vi "Process.vi"(8 "error in":errorcluster, 11 "Instrument.Example":refnum<class "Instrument.OxfordVRM.lvclass">) -> (0 "error out":errorcluster, 3 "Instrument.Example out":refnum<class "Instrument.OxfordVRM.lvclass">)   [LabVIEW 2019, in "Instrument.OxfordVRM.lvclass"]
doc: "---------------------------------------------------------------\nJKI State Machine Objects™\nhttp://jki.net/state-machine-objects/\nCopyright (C) 2005-2015, JKI <info@jki.net>\nALL RIGHTS RESERVED"
uses:
  Instrument.OxfordVRM.lvclass
  C:/Program Files (x86)/National Instruments/LabVIEW 2019/vi.lib/JKI/JKI SMO/SMO/SMO.lvclass
  C:/Program Files (x86)/National Instruments/LabVIEW 2019/user.lib/LevyLab/Instrument Framework/Instrument/Instrument.lvclass
  Typedefs/VRM Magnet Axis--Enum.ctl
  Instrument.OxfordVRM.lvclass/Instrument.OxfordVRM.ctl
  <vilib>/JKI/JKI SMO/SMO/SMO.lvclass/SMO.ctl
  <vilib>/JKI/JKI SMO/SMO/Private/ReftoDVR--SMO.vi
  <userlib>/LevyLab/Instrument Framework/Instrument Types/Cryostat/Instrument.Cryostat.lvclass
  <vilib>/JKI/JKI SMO/SMO/SMO.lvclass
  <userlib>/LevyLab/Instrument Framework/Instrument/Instrument.lvclass
  <userlib>/LevyLab/Debug/Debug.lvlib
panel:
  out "State":string
  out "timer":u32
  # "For instructions on how to use the JKI State Machine Objects, examples and video tutorials, visit:\nhttp://jki.net/state-machine-objects/\n\nJKI State Machine Objects™\nhttp://jki.net/state-machine-objects/\nCopyright (C) 2005-2015, JKI <info@jki.net>\nALL RIGHTS RESERVED"
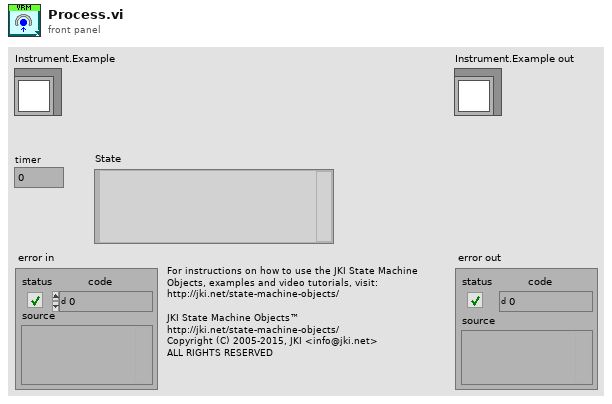
[diagram p1: front panel]
types:
  T1 = enum32{"invalid app kind", "Development System", "Run Time System", "Student Edition", "Embedded LabVIEW", "Evaluation", "Custom"}
  T2 = enum32{"Invalid", "Standard", "Closed", "Hidden", "Minimized", "Maximized"}
  T3 = typedef "Instrument.OxfordVRM.lvclass/VRM Magnet Axis--Enum.ctl" = enum16{"X", "Y", "Z", "ALL"}
  T4 = cluster{"Core":cluster{"Current VI Reference":refnum<vi>, "Close Panel on Exit?":bool, "Last Error":cluster{"error":errorcluster, "previous state":string, "remaining states":string}, "Shutdown?":bool}, "SelfRef":refnum<class "Instrument.OxfordVRM.lvclass">, "Field (T)":dbl[], "Field Rate (T/min)":dbl, "Axis":T3, "Running Step":i32, "sequence":string[]}
  T5 = cluster{"Current VI Reference":refnum<vi>, "Close Panel on Exit?":bool, "Last Error":cluster{"error":errorcluster, "previous state":string, "remaining states":string}, "Shutdown?":bool}
  T6 = typedef "Instrument.OxfordVRM.lvclass/getAll.ctl" = cluster{"Field":dbl[], "Target Field":dbl[], "Target Field Rate":dbl[], "PSU Current":dbl[], "PSU Voltage":dbl[], "Status":string[]}
  T7 = typedef "Debug.lvlib/Attribute.Debug.lvclass/DebugBehavior.ctl" = enum16{"Normal", "Debug"}
  T8 = typedef "SMO.lvclass/Protected Events.ctl" = cluster{"StopProcesses":refnum<user-event>, "AbortProcesses":refnum<user-event>, "Config Changed":refnum<user-event>, "Dependency":refnum<user-event>}
  T9 = typedef "Instrument.OxfordVRM.lvclass/PrivateEvents--Cluster.ctl" = cluster{"SequenceSetMagnetField":refnum<user-event>, "AbortSequence":refnum<user-event>}
  T10 = cluster{"Holding":bool, "Ramp to Setpoint":bool, "Ramp to Zero":bool, "Clamp":bool}
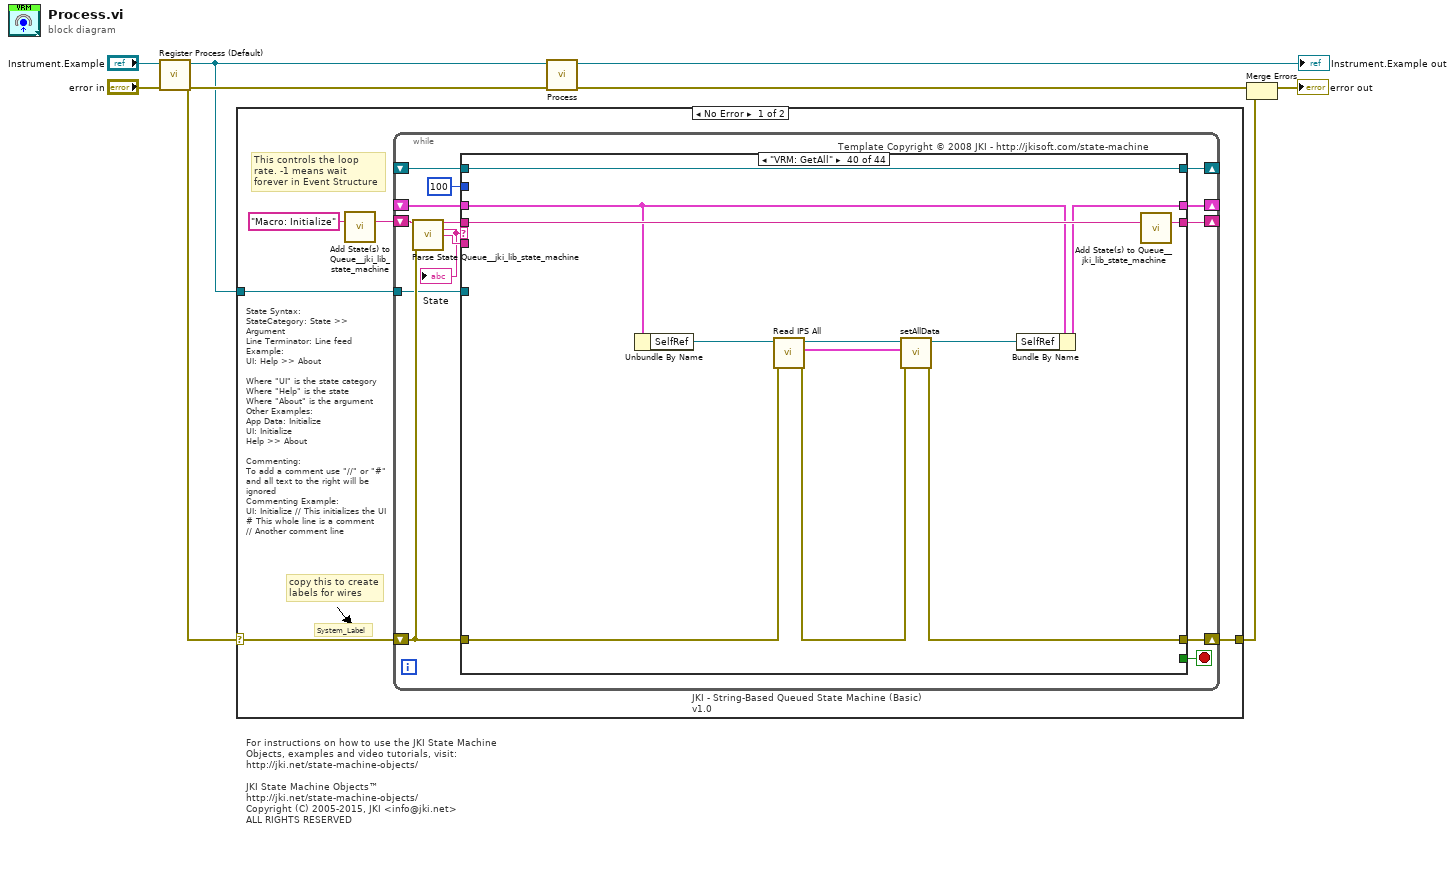
[diagram p0: block diagram]
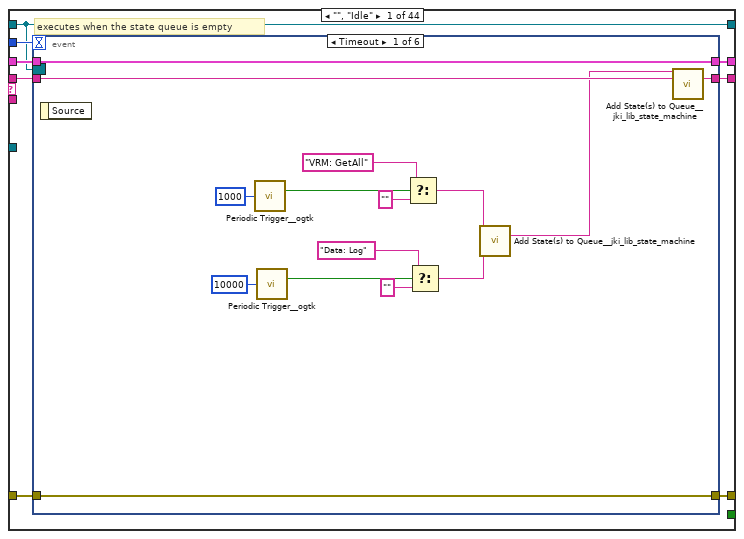
[diagram p2: hidden frame]
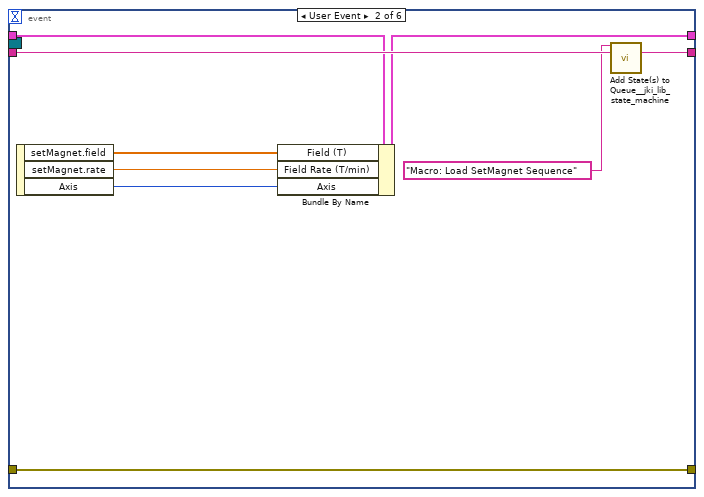
[diagram p3: hidden frame]
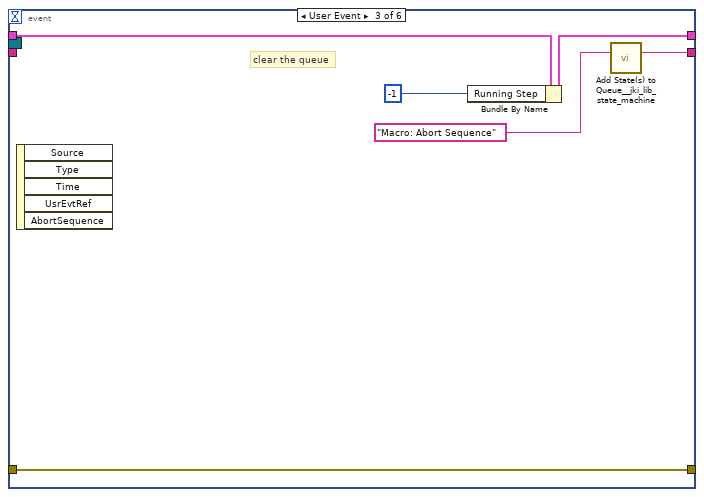
[diagram p4: hidden frame]
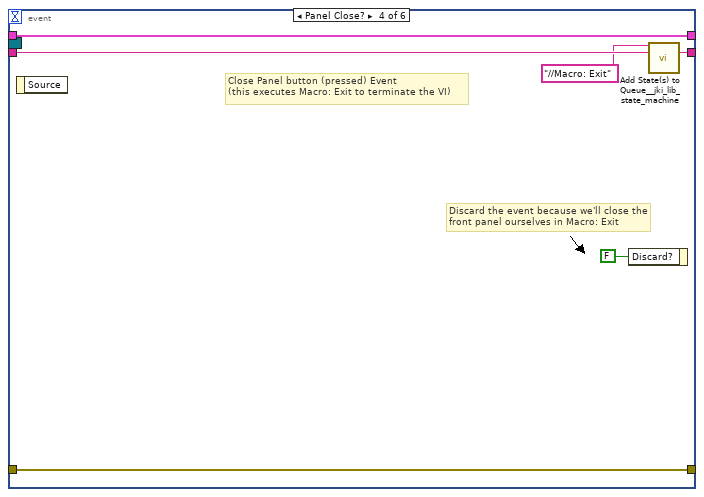
[diagram p5: hidden frame]
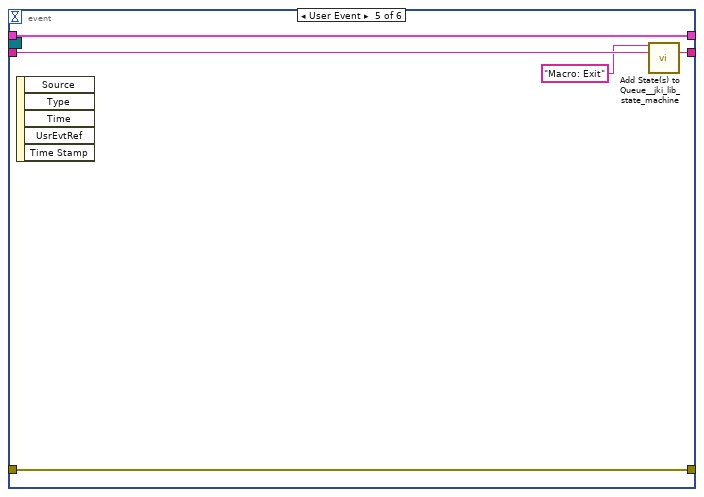
[diagram p6: hidden frame]
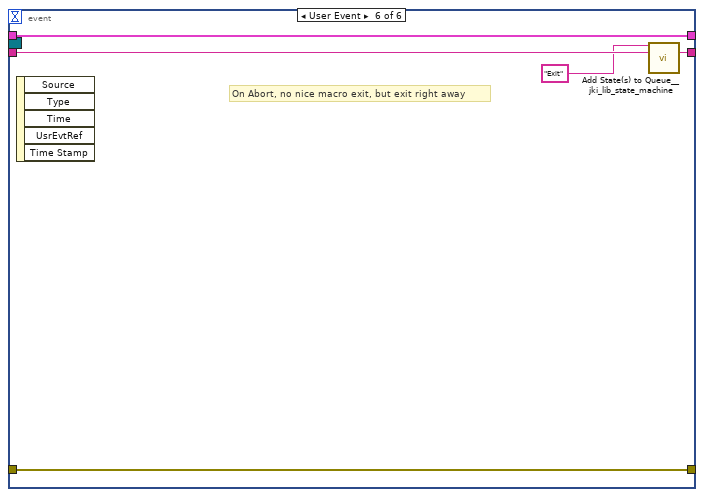
[diagram p7: hidden frame]
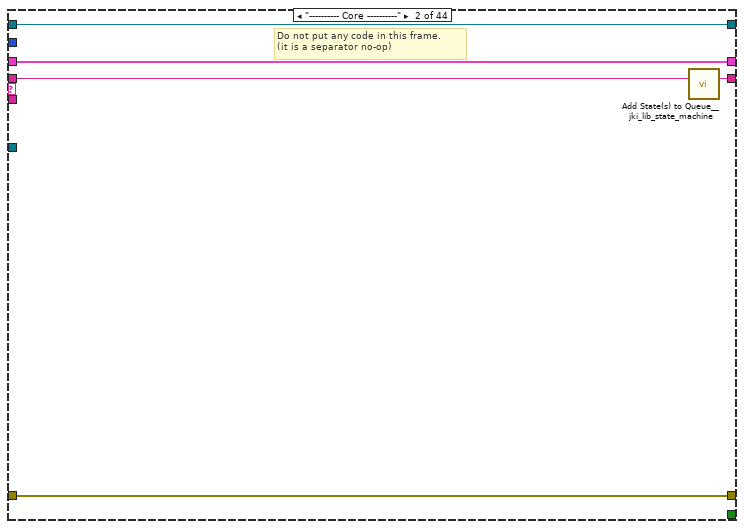
[diagram p8: hidden frame]
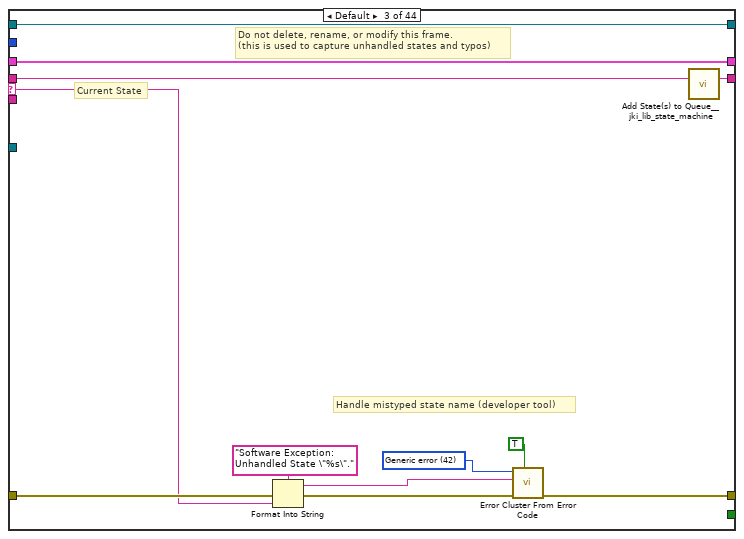
[diagram p9: hidden frame]
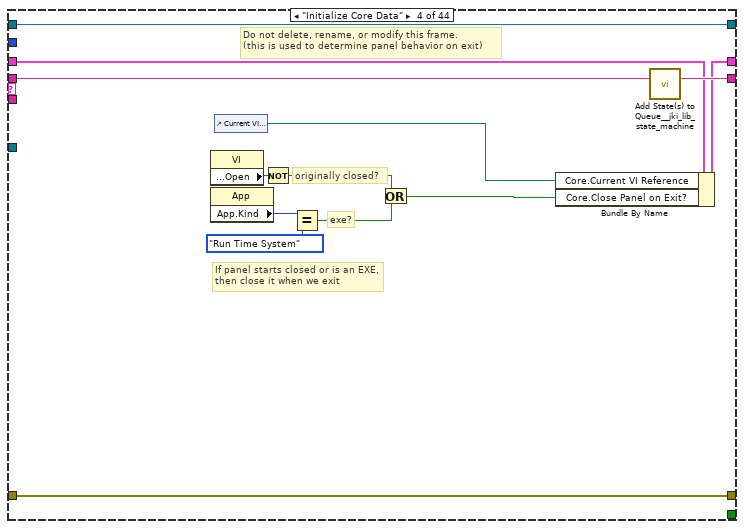
[diagram p10: hidden frame]
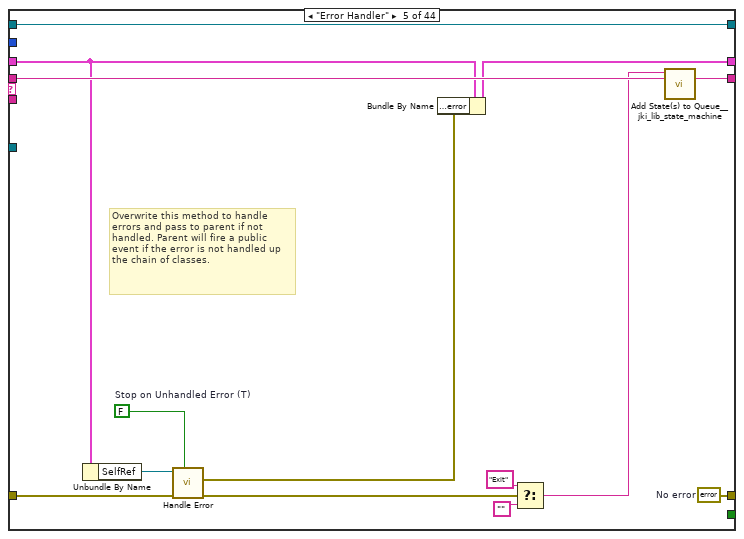
[diagram p11: hidden frame]
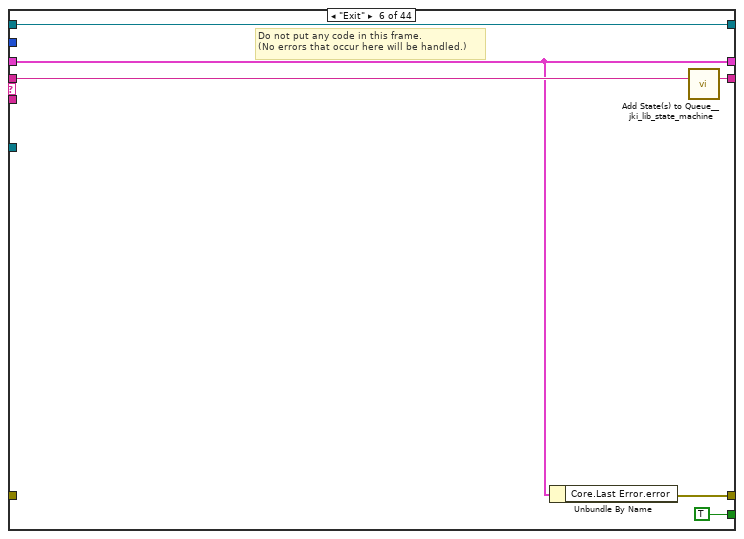
[diagram p12: hidden frame]
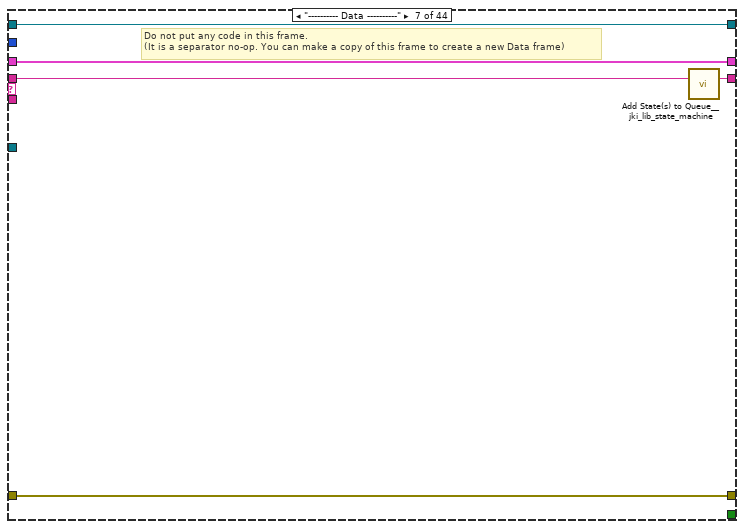
[diagram p13: hidden frame]
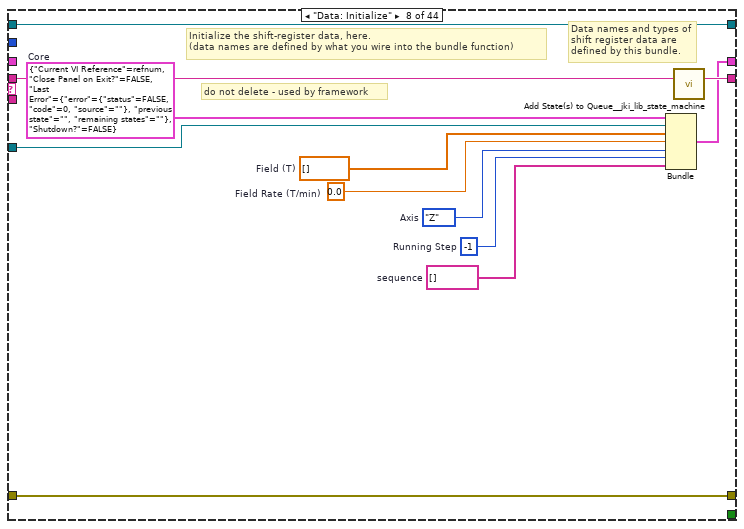
[diagram p14: hidden frame]
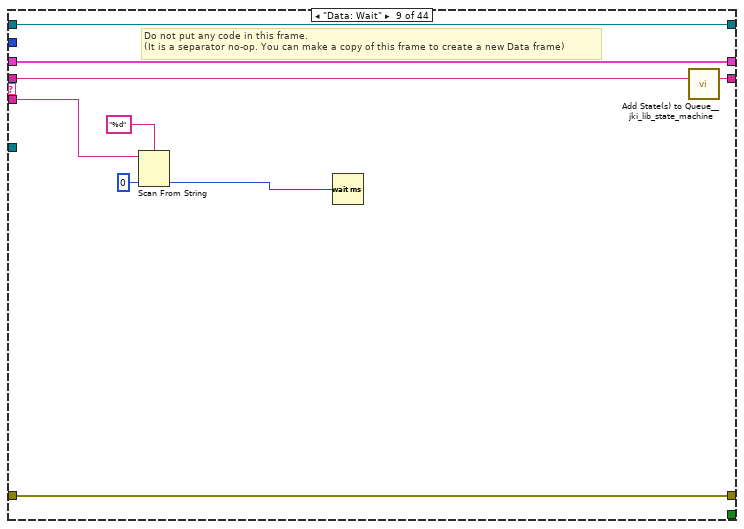
[diagram p15: hidden frame]
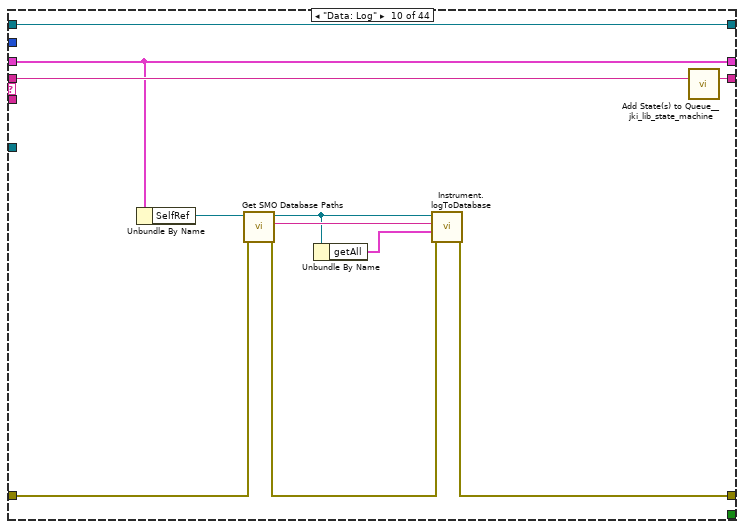
[diagram p16: hidden frame]
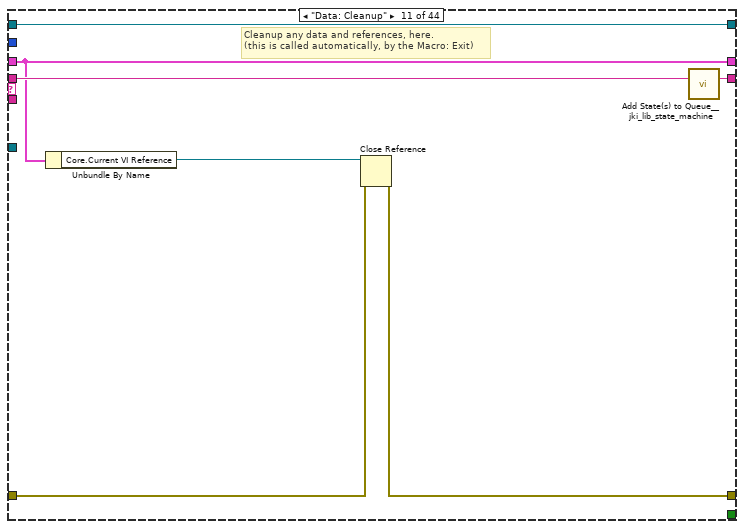
[diagram p17: hidden frame]
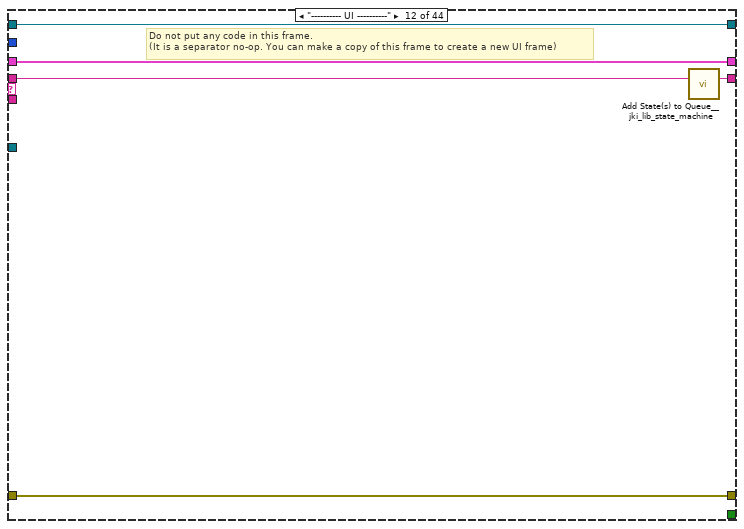
[diagram p18: hidden frame]
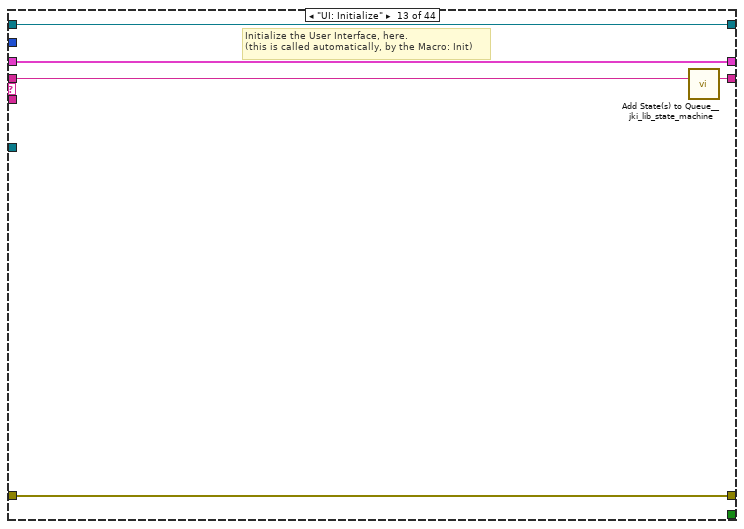
[diagram p19: hidden frame]
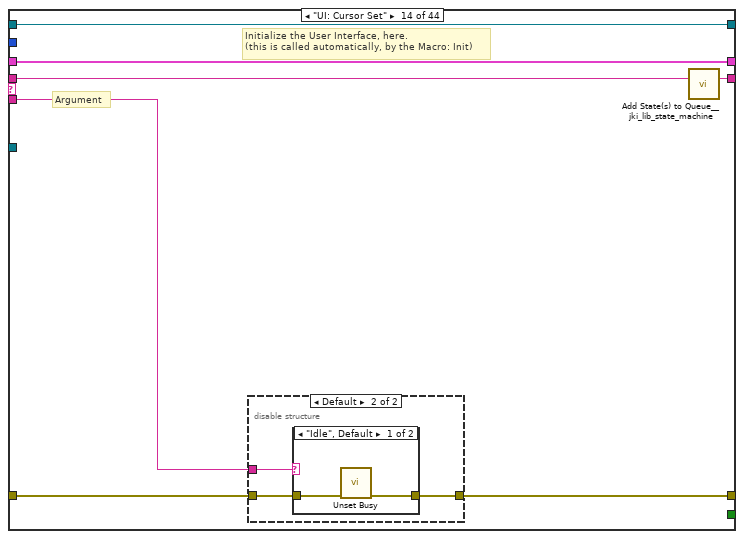
[diagram p20: hidden frame]
diagram:
  # "For instructions on how to use the JKI State Machine Objects, examples and video tutorials, visit:\nhttp://jki.net/state-machine-objects/\n\nJKI State Machine Objects™\nhttp://jki.net/state-machine-objects/\nCopyright (C) 2005-2015, JKI <info@jki.net>\nALL RIGHTS RESERVED"
  n1 = call <vilib>:"Register Process (Default).vi"("error in (no error)"="error in", "SMO"="Instrument.Example") -> ("error out"=w5:errorcluster, "SelfRef"=w4:refnum<class "Instrument.OxfordVRM.lvclass">)  [unwired: 8 in]
  n2 = case shown="No Error" w5 {
    selector: w5 -> [w10 w673]
    tunnel: w4 -> [w11 _]
    tunnel: [w9 w673] -> w1
    frame No Error {
      # "State Syntax:\nStateCategory: State >> Argument\nLine Terminator: Line feed\nExample:\nUI: Help >> About\n\nWhere \"UI\" is the state category\nWhere \"Help\" is the state\nWhere \"About\" is the argument\nOther Examples:\nApp Data: Initialize\nUI: Initialize\nHelp >> About\n\nCommenting:\nTo add a comment use \"//\" or \"#\" and all text to the right will be ignored\nCommenting Example:\nUI: Initialize // This initializes the UI\n# This whole line is a comment\n// Another comment line"
      # "copy this to create labels for wires"
      # "This controls the loop rate. -1 means wait forever in Event Structure"
      # "System_Label"
      n3 = call <vilib>:"Add State(s) to Queue__jki_lib_state_machine.vi"("State(s) in (\"\")"="Macro: Initialize") -> ("States Out"=w13:string)  [unwired: 14 in]
      n4 = while "JKI - String-Based Queued State Machine (Basic) v1.0" {
        shift-right: [w21] -> _
        shift-left: _ -> [w20]
        shift-right: [w24] -> w9
        shift-left: w10 -> [w18]
        shift-right: [w23] -> _
        shift-left: w13 -> [w25]
        tunnel: w11 -> [w17]
        shift-right: [w16] -> _
        shift-left: _ -> [w15]
        stop <- w22 stop-if-true
        # "Template Copyright © 2008 JKI - http://jkisoft.com/state-machine"
        n5 = call <vilib>:"Parse State Queue__jki_lib_state_machine.vi"("State Queue"=w25, "Error In (no error)"=w18) -> ("Remaining States"=w27:string, "Current State"=w14:string, "Arguments"=w26:string)  [unwired: 11 in]
        "State" <- w14
        n6 = case shown="\"VRM: GetAll\"" w14 {
          selector: w14 -> [_ _ w88 _ _ _ _ _ _ _ _ _ _ _ _ _ _ _ _ _ _ _ _ _ _ _ _ _ _ w429 _ w471 w493 w515 w538 w562 _ _ _ _ w616 w631 w647 w664]
          tunnel: w27 -> [w35 w86 w92 w111 w125 w131 w136 w148 w157 w168 w175 w180 w185 w192 w208 w240 w249 w264 w285 w302 _ _ w361 w372 w377 w390 w396 w405 w412 w441 w459 w481 w503 w525 w548 w571 w580 w589 w598 w610 w625 w640 w655 w672]
          tunnel: w26 -> [_ _ _ _ _ _ _ _ w149 _ _ _ _ w186 w202 _ _ _ _ _ _ _ _ _ _ _ _ _ _ w430 w452 _ _ _ _ _ _ _ _ _ _ _ _ _]
          tunnel: w20 -> [w33 w83 w90 w102 w119 w127 w133 _ w154 w165 w170 w177 w183 w190 w204 w237 w246 w252 w270 w290 w312 w350 w358 w362 w374 w388 w394 w397 w408 w415 w451 w474 w496 w518 w545 w568 w574 w586 w595 w605 w622 w637 w652 w669]
          tunnel: [w32 w84 w94 w108 w120 w126 w134 w137 w155 w158 w171 w178 w182 w187 w205 w238 w241 w251 w283 w300 w309 w349 w359 w364 w375 w383 w392 w402 w409 w419 w454 w463 w485 w507 w530 w561 w577 w583 w592 w599 w619 w634 w643 w659] -> w24
          tunnel: w18 -> [w31 w84 w93 w108 w121 _ w134 w137 w155 w159 w172 w178 w182 w188 w206 w238 w241 w250 w283 w300 w310 w349 w359 w365 w375 w384 w392 w402 w409 w418 w455 w462 w484 w506 w532 w556 w577 w582 w591 w604 w613 w629 w644 w660]
          tunnel: [w34 w85 w91 w110 w124 w130 w135 w147 w156 w167 w174 w179 w184 w191 w207 w239 w248 w263 w284 w301 w318 w356 w360 w371 w376 w389 w395 w404 w411 w440 w458 w480 w502 w524 w547 w570 w579 w588 w597 w609 w624 w639 w654 w671] -> w23
          tunnel: [_ _ _ _ _ TRUE _ _ _ _ _ _ _ _ _ _ _ _ _ _ _ _ _ _ _ _ _ _ _ _ _ _ _ _ _ _ _ _ _ _ _ _ _ _] -> w22
          tunnel: [w30 w83 w90 w109 w118 w127 w133 w146 w154 w165 w170 w177 w183 w190 w204 w237 w246 w253 w271 w298 w313 w351 w358 w362 w374 w388 w394 w399 w407 w413 w450 w473 w495 w517 w544 w567 w573 w581 w590 w606 w621 w636 w651 w668] -> w21
          tunnel: 100 ("Timeout") -> [w29 _ _ _ _ _ _ _ _ _ _ _ _ _ _ _ _ _ _ _ _ _ _ _ _ _ _ _ _ _ _ _ _ _ _ _ _ _ _ _ _ _ _ _]
          tunnel: w17 -> [_ _ _ _ _ _ _ w138 _ _ _ _ _ _ _ _ _ _ _ _ _ _ _ _ _ _ _ _ _ _ _ _ _ _ _ _ _ _ _ _ _ _ _ _]
          tunnel: [w28 w82 w87 w99 w123 w128 w132 w145 w153 w166 w169 w176 w181 w189 w201 w236 w247 w262 w277 w299 w317 w355 w357 w370 w373 w387 w393 w403 w410 w439 w457 w479 w501 w523 w546 w569 w578 w587 w596 w608 w623 w638 w653 w670] -> w16
          tunnel: w15 -> [w28 w82 w87 w99 w123 w128 w132 w145 w153 w166 w169 w176 w181 w189 w201 w236 w247 w262 w277 w299 w317 w355 w357 w370 w373 _ w393 w403 w410 w439 w457 w479 w501 w523 w546 w569 w578 w587 w596 w608 w623 w638 w653 w670]
          frame "", "Idle" {
            # "executes when the state queue is empty"
            n7 = event shown="[0] Timeout" {
              selector: w28 -> [_ _ _ _ _ _]
              dyn-events: _ -> [_ _ _ _ _ _]
              timeout: w29 -> [_ _ _ _ _ _]
              tunnel: w35 -> [w50 w57 _ w71 w76 w81]
              tunnel: [w49 w58 w64 w70 w75 w80] -> w34
              tunnel: w33 -> [w47 w55 w62 w68 w73 w78]
              tunnel: [w48 w59 w65 w69 w74 w79] -> w32
              tunnel: w31 -> [w48 w59 w65 w69 w74 w79]
              tunnel: [w47 w54 w61 w68 w73 w78] -> w30
              event Timeout {
                n8 = event-data() -> ()  [unwired: 1 in, 1 out]
                n9 = call <userlib>:"Periodic Trigger__ogtk.vi"("time (ms)"=u32 1000) -> ("Triggered"=w45:bool)  [unwired: 12 in, 2 out]
                n10 = call <userlib>:"Periodic Trigger__ogtk.vi"("time (ms)"=u32 10000) -> ("Triggered"=w40:bool)  [unwired: 12 in, 2 out]
                n11 = Select(t="VRM: GetAll" ("State(s) in Front (\"\")"), s=w45, f="") -> (s? t:f=w37:string)
                n12 = Select(t="Data: Log" ("State(s) in Front (\"\")"), s=w40, f="") -> (s? t:f=w38:string)
                n13 = call <vilib>:"Add State(s) to Queue__jki_lib_state_machine.vi"("State(s) in Front (\"\")"=w37, "State(s) at Back (\"\")"=w38) -> ("States Out"=w36:string)  [unwired: 13 in]
                n14 = call <vilib>:"Add State(s) to Queue__jki_lib_state_machine.vi"("State(s) in Front (\"\")"=w36, "State(s) in (\"\")"=w50) -> ("States Out"=w49:string)  [unwired: 13 in]
              }
              event User Event {
                n15 = event-data() -> ("setMagnet.field"=w56:dbl[], "setMagnet.rate"=w52:dbl, "Axis"=w51:T3)  [unwired: 1 in]
                n16 = Bundle By Name(cluster=w55, "Field (T)"=w56, "Field Rate (T/min)"=w52, "Axis"=w51) -> (w54:T4)
                n17 = call <vilib>:"Add State(s) to Queue__jki_lib_state_machine.vi"("State(s) in Front (\"\")"="Macro: Load SetMagnet Sequence" ("State(s) at Back (\"\")"), "State(s) in (\"\")"=w57) -> ("States Out"=w58:string)  [unwired: 13 in]
              }
              event User Event {
                # "clear the queue"
                n18 = event-data() -> ()  [unwired: 1 in, 5 out]
                n19 = Bundle By Name(cluster=w62, "Running Step"=-1) -> (w61:T4)
                n20 = call <vilib>:"Add State(s) to Queue__jki_lib_state_machine.vi"("State(s) in (\"\")"="Macro: Abort Sequence" ("State(s) at Back (\"\")")) -> ("States Out"=w64:string)  [unwired: 14 in]
              }
              event Panel Close? {
                # "Discard the event because we'll close the front panel ourselves in Macro: Exit"
                # "Close Panel button (pressed) Event\n(this executes Macro: Exit to terminate the VI)"
                n21 = event-data() -> ()  [unwired: 1 in, 1 out]
                n22 = event-data("Discard?"=FALSE) -> ()  [unwired: 1 in, 1 out]
                n23 = call <vilib>:"Add State(s) to Queue__jki_lib_state_machine.vi"("State(s) in Front (\"\")"="//Macro: Exit", "State(s) in (\"\")"=w71) -> ("States Out"=w70:string)  [unwired: 13 in]
              }
              event User Event {
                n24 = event-data() -> ()  [unwired: 1 in, 5 out]
                n25 = call <vilib>:"Add State(s) to Queue__jki_lib_state_machine.vi"("State(s) in Front (\"\")"="Macro: Exit", "State(s) in (\"\")"=w76) -> ("States Out"=w75:string)  [unwired: 13 in]
              }
              event User Event {
                # "On Abort, no nice macro exit, but exit right away"
                n26 = event-data() -> ()  [unwired: 1 in, 5 out]
                n27 = call <vilib>:"Add State(s) to Queue__jki_lib_state_machine.vi"("State(s) in Front (\"\")"="Exit", "State(s) in (\"\")"=w81) -> ("States Out"=w80:string)  [unwired: 13 in]
              }
            }
          }
          frame "---------- Core ----------" {
            # "Do not put any code in this frame.\n(it is a separator no-op)"
            n28 = call <vilib>:"Add State(s) to Queue__jki_lib_state_machine.vi"("State(s) in (\"\")"=w86) -> ("States Out"=w85:string)  [unwired: 14 in]
          }
          frame Default {
            w97 = 42 items=["No error", "Argument error", "Memory is full", "Out of zone", "End of file", "File already open", "Generic file I/O error", "File not found", "File permission error", "Disk is full", "Duplicate path", "Too many files open", "System feature not enabled", "Resource file not found", "Cannot add resource", "Resource not found", "Image not found", "Image memory error", "Pen does not exist", "Config type invalid", "Config token not found", "Config parse error", "Config memory error", "Bad external code format", "Bad external code offset", "External code not present", "Null window", "Destroy window error", "Null menu", "Print aborted", "Bad print record", "Print driver error", "Windows error during printing", "Memory error during printing", "Print dialog error", "Generic print error", "Invalid device refnum", "Device not found", "Device parameter error", "Device unit error", "Cannot open device", "Device call aborted", "Generic error", "Cancelled by user", "Object ID too low", "Object ID too high", "Object not in heap", "Unknown heap", "Unknown object (invalid DefProc)", "Unknown object (DefProc not in table)", "Message out of range", "Invalid (null) method", "Unknown message", "Manager call not supported", "Bad address", "Network operation in progress", "Network operation timed out", "Connection is busy", "Network attribute not supported", "Network error", "Address in use", "System out of memory", "Connection aborted", "Connection refused", "Not connected", "Already connected", "Connection closed", "Initialization error (interapplication manager)", "Bad occurrence", "Wait on unbound occurrence handler", "Occurrence queue overflow", "Datalog type conflict", "Unused", "Unrecognized type (interapplication manager)", "Memory corrupt", "Failed to make temporary DLL", "Old CIN version", "Drag socket not found", "Failed to load drop-object", "Failed to register OLE object", "Failed to release OLE object", "Format specifier type mismatch", "Unknown format specifier", "Too few format specifiers", "Too many format specifiers", "Scan failed", "Newer CIN version", "Error converting to variant", "Runtime menu error", "Password tampered", "Variant attribute not found", "Incompatible variant data type", "Event data is not available", "Event Store is not present", "Occurrence is not found", "Event Queue is not created", "Event info is not available", "Refnum passed is NULL", "Error retrieving Class GUID", "Error retrieving CoClass GUID", "Error retrieving TypeLib GUID.", "Bad built application magic bytes.", "Specific driver is different from the specific driver associated with the Logical Name.", "There is no session opened to the class driver.", "Max Error", "MAX - Error with config objects", "MAX - Error loading configuration", "MAX - Group not supported"]
            # "Current State"
            # "Do not delete, rename, or modify this frame.\n(this is used to capture unhandled states and typos)"
            # "Handle mistyped state name (developer tool)"
            n29 = Format Into String(format string="Software Exception: Unhandled State \"%s\"." ("message"), error in=w93, w88) -> (resulting string=w96:string, error out=w95:errorcluster)  [unwired: 1 in]
            n30 = call <vilib>:"Error Cluster From Error Code.vi"("show call chain? (False)"=TRUE, "error in (no error)"=w95, "error message (\"\")"=w96, "error code (0)"=w97) -> ("error out"=w94:errorcluster)  [unwired: 5 in]
            n31 = call <vilib>:"Add State(s) to Queue__jki_lib_state_machine.vi"("State(s) in (\"\")"=w92) -> ("States Out"=w91:string)  [unwired: 14 in]
          }
          frame "Initialize Core Data" {
            # "Do not delete, rename, or modify this frame.\n(this is used to determine panel behavior on exit)"
            # "originally closed?"
            # "exe?"
            # "If panel starts closed or is an EXE, then close it when we exit"
            n32 = property class="VI"() -> ("Front Panel.Open"=w107:bool)  [unwired: 2 in, 2 out]
            n33 = property class="App"() -> ("App.Kind"=w106:T1)  [unwired: 2 in, 2 out]
            n34 = control-ref of="Current VI Reference"() -> (w100:refnum<vi>)
            n35 = Not(x=w107) -> (.not. x?=w104:bool)
            n36 = Equal?(x=w106, y=T1."Run Time System" ("Application:Kind")) -> (x = y?=w103:bool)
            n37 = Or(x=w104, y=w103) -> (x .or. y?=w101:bool)
            n38 = Bundle By Name(cluster=w102, "Core.Current VI Reference"=w100, "Core.Close Panel on Exit?"=w101) -> (w109:T4)
            n39 = call <vilib>:"Add State(s) to Queue__jki_lib_state_machine.vi"("State(s) in (\"\")"=w111) -> ("States Out"=w110:string)  [unwired: 14 in]
          }
          frame "Error Handler" {
            w112 = FALSE  # Stop on Unhandled Error (T)
            w120 = errorcluster {"status"=FALSE, "code"=0, "source"=""}  # No error
            # "Overwrite this method to handle errors and pass to parent if not handled. Parent will fire a public event if the error is not handled up the chain of classes."
            n40 = Unbundle By Name(w119) -> ("SelfRef"=w122:refnum<class "Instrument.OxfordVRM.lvclass">)
            n41 = call-dynamic "Handle Error.vi"("Stop on Unhandled Error (T)"=w112, "error in"=w121, "SMO"=w122) -> ("handling error"=w113:errorcluster, "Unhandled error"=w116:errorcluster)  [unwired: 6 in, 1 out]
            n42 = Bundle By Name(cluster=w119, "Core.Last Error.error"=w116) -> (w118:T4)
            n43 = Select(t="Exit", s=w113, f="") -> (s? t:f=w117:string)
            n44 = call <vilib>:"Add State(s) to Queue__jki_lib_state_machine.vi"("State(s) in Front (\"\")"=w117, "State(s) in (\"\")"=w125) -> ("States Out"=w124:string)  [unwired: 13 in]
          }
          frame "Exit" {
            # "Do not put any code in this frame.\n(No errors that occur here will be handled.)"
            n45 = Unbundle By Name(w127) -> ("Core.Last Error.error"=w126:errorcluster)
            n46 = call <vilib>:"Add State(s) to Queue__jki_lib_state_machine.vi"("State(s) in (\"\")"=w131) -> ("States Out"=w130:string)  [unwired: 14 in]
          }
          frame "---------- Data ----------" {
            # "Do not put any code in this frame.\n(It is a separator no-op. You can make a copy of this frame to create a new Data frame)"
            n47 = call <vilib>:"Add State(s) to Queue__jki_lib_state_machine.vi"("State(s) in (\"\")"=w136) -> ("States Out"=w135:string)  [unwired: 14 in]
          }
          frame "Data: Initialize" {
            w139 = T5 {"Current VI Reference"=refnum, "Close Panel on Exit?"=FALSE, "Last Error"={"error"={"status"=FALSE, "code"=0, "source"=""}, "previous state"="", "remaining states"=""}, "Shutdown?"=FALSE}  # Core
            w140 = VRM_Magnet_Axis--Enum."Z"  # Axis
            w141 = string[] []  # sequence
            w142 = -1  # Running Step
            w143 = 0.0  # Field Rate (T/min)
            w144 = dbl[] []  # Field (T)
            # "do not delete - used by framework"
            # "Data names and types of shift register data are defined by this bundle."
            # "Initialize the shift-register data, here.\n(data names are defined by what you wire into the bundle function)"
            n48 = Bundle("Core"=w139, "SelfRef"=w138, "Field (T)"=w144, "Field Rate (T/min)"=w143, "Axis"=w140, "Running Step"=w142, "sequence"=w141) -> (w146:T4)  [unwired: 1 in]
            n49 = call <vilib>:"Add State(s) to Queue__jki_lib_state_machine.vi"("State(s) in (\"\")"=w148) -> ("States Out"=w147:string)  [unwired: 14 in]
          }
          frame "Data: Wait" {
            # "Do not put any code in this frame.\n(It is a separator no-op. You can make a copy of this frame to create a new Data frame)"
            n50 = Scan From String(format string="%d", input string=w149, default 1=u32 0 ("default value 1")) -> (output 1=w150:u32)  [unwired: 2 in, 3 out]
            n51 = Wait (ms)(milliseconds to wait=w150) -> ()  [unwired: 1 out]
            n52 = call <vilib>:"Add State(s) to Queue__jki_lib_state_machine.vi"("State(s) in (\"\")"=w157) -> ("States Out"=w156:string)  [unwired: 14 in]
          }
          frame "Data: Log" {
            n53 = Unbundle By Name(w165) -> ("SelfRef"=w164:refnum<class "Instrument.OxfordVRM.lvclass">)
            n54 = call-dynamic "Get SMO Database Paths.vi"("error in (no error)"=w159, "Instrument.VRM in"=w164) -> ("error out"=w160:errorcluster, "Paths"=w163:string, "Instrument.VRM out"=w162:refnum<class "Instrument.OxfordVRM.lvclass">)  [unwired: 7 in]
            n55 = Unbundle By Name(w162) -> ("getAll"=w161:T6)
            n56 = call <userlib>:"Instrument.logToDatabase.vi"("error in (no error)"=w160, "Data"=w161, "Paths"=w163, "Instrument"=w162) -> ("error out"=w158:errorcluster)  [unwired: 6 in, 1 out]
            n57 = call <vilib>:"Add State(s) to Queue__jki_lib_state_machine.vi"("State(s) in (\"\")"=w168) -> ("States Out"=w167:string)  [unwired: 14 in]
          }
          frame "Data: Cleanup" {
            # "Cleanup any data and references, here.\n(this is called automatically, by the Macro: Exit)"
            n58 = Unbundle By Name(w170) -> ("Core.Current VI Reference"=w173:refnum<vi>)
            n59 = Close Reference(reference=w173, error in (no error)=w172) -> (error out=w171:errorcluster)
            n60 = call <vilib>:"Add State(s) to Queue__jki_lib_state_machine.vi"("State(s) in (\"\")"=w175) -> ("States Out"=w174:string)  [unwired: 14 in]
          }
          frame "---------- UI ----------" {
            # "Do not put any code in this frame.\n(It is a separator no-op. You can make a copy of this frame to create a new UI frame)"
            n61 = call <vilib>:"Add State(s) to Queue__jki_lib_state_machine.vi"("State(s) in (\"\")"=w180) -> ("States Out"=w179:string)  [unwired: 14 in]
          }
          frame "UI: Initialize" {
            # "Initialize the User Interface, here.\n(this is called automatically, by the Macro: Init)"
            n62 = call <vilib>:"Add State(s) to Queue__jki_lib_state_machine.vi"("State(s) in (\"\")"=w185) -> ("States Out"=w184:string)  [unwired: 14 in]
          }
          frame "UI: Cursor Set" {
            # "Argument"
            # "Initialize the User Interface, here.\n(this is called automatically, by the Macro: Init)"
            n63 = disable-structure shown="Default" {
              disable-tunnel: w188 -> [w193 w196]
              disable-tunnel: [w193 w195] -> w187
              disable-tunnel: w186 -> [_ w194]
              frame condition #0 {
              }
              frame condition #1 (active) {
                n64 = case shown="\"Idle\", Default" w194 {
                  tunnel: w196 -> [w198 w200]
                  tunnel: [w197 w199] -> w195
                  frame "Idle", Default {
                    n65 = call <vilib>:"Unset Busy.vi"("error in (no error)"=w198) -> ("error out"=w197:errorcluster)  [unwired: 10 in]
                  }
                  frame "Busy" {
                    n66 = call <vilib>:"Set Busy.vi"("error in (no error)"=w200) -> ("error out"=w199:errorcluster)  [unwired: 9 in, 1 out]
                  }
                }
              }
            }
            n67 = call <vilib>:"Add State(s) to Queue__jki_lib_state_machine.vi"("State(s) in (\"\")"=w192) -> ("States Out"=w191:string)  [unwired: 14 in]
          }
          frame "UI: Front Panel State" {
            # "Argument"
            # "Set Front Panel Open or Closed\n(Usage: \"UI: Front Panel State >> Open|Close\")"
            n68 = Unbundle By Name(w204) -> ("Core.Current VI Reference"=w203:refnum<vi>)
            n69 = disable-structure shown="Default" {
              disable-tunnel: w206 -> [w212 w235]
              disable-tunnel: [w211 w235] -> w205
              disable-tunnel: w203 -> [w210 _]
              disable-tunnel: w202 -> [w209 _]
              frame condition #0 (active) {
                n70 = case shown="\"Close\"" w209 {
                  tunnel: w212 -> [w216 w229]
                  tunnel: [w218 w230] -> w211
                  tunnel: w210 -> [w217 w227]
                  frame "Open", Default {
                    n71 = property class="VI"(reference=w217, error in=w216) -> (reference out=w214:refnum<vi>, error out=w215:errorcluster, "FP.State"=w213:T2)
                    n72 = case shown="\"Closed\"" w213 {
                      tunnel: [w221 w224] -> w218
                      tunnel: w215 -> [w220 w224]
                      tunnel: w214 -> [w219 _]
                      frame "Closed" {
                        n73 = invoke class="VI" method="FP.Open"(reference=w219, error in=w220, "Activate"=TRUE, "State"=T2."Standard") -> (error out=w221:errorcluster)  [unwired: 1 in, 4 out]
                      }
                      frame Default {
                      }
                    }
                  }
                  frame "Close" {
                    n74 = property class="VI"(reference=w227, error in=w229) -> (reference out=w226:refnum<vi>, error out=w228:errorcluster, "FP.State"=w225:T2)
                    n75 = case shown="Default" w225 {
                      tunnel: [w231 w234] -> w230
                      tunnel: w228 -> [w231 w233]
                      tunnel: w226 -> [_ w232]
                      frame "Invalid", "Closed" {
                      }
                      frame Default {
                        n76 = invoke class="VI" method="FP.Close"(reference=w232, error in=w233) -> (error out=w234:errorcluster)  [unwired: 1 in, 2 out]
                      }
                    }
                  }
                }
              }
              frame condition #1 {
              }
            }
            n77 = call <vilib>:"Add State(s) to Queue__jki_lib_state_machine.vi"("State(s) in (\"\")"=w208) -> ("States Out"=w207:string)  [unwired: 14 in]
          }
          frame "---------- Macro ----------" {
            # "Do not put any code in this frame.\n(It is a separator no-op. You can make a copy of this frame to create a new Macro frame)"
            n78 = call <vilib>:"Add State(s) to Queue__jki_lib_state_machine.vi"("State(s) in (\"\")"=w240) -> ("States Out"=w239:string)  [unwired: 14 in]
          }
          frame "Macro: Initialize" {
            # "Initialization Macro\n(This is called once, when the VI starts)"
            n79 = call <vilib>:"Add State(s) to Queue__jki_lib_state_machine.vi"("State(s) in Front (\"\")"="Data: Initialize\nInitialize Core Data\nEvents: Register", "State(s) in (\"\")"="Process: Sync", "State(s) at Back (\"\")"="UI: Initialize\nUI: Front Panel State >> Close\nMacro: Debug\nVRM: Open\nVRM: GetAll") -> ("States Out"=w244:string)  [unwired: 12 in]
            n80 = call <vilib>:"Add State(s) to Queue__jki_lib_state_machine.vi"("State(s) in Front (\"\")"=w244, "State(s) in (\"\")"=w249) -> ("States Out"=w248:string)  [unwired: 13 in]
          }
          frame "Macro: Debug" {
            # "exe?"
            # "If pane is an EXE, then close it when we exit"
            # "Macro: Debug\n(get debug behavior, determine UI and determine shutdown behavior)"
            n81 = Unbundle By Name(w252) -> ("Core.Close Panel on Exit?"=w256:bool, "SelfRef"=w261:refnum<class "Instrument.OxfordVRM.lvclass">)
            n82 = property class="App"() -> ("App.Kind"=w259:T1)  [unwired: 2 in, 2 out]
            n83 = Equal?(x=w259, y=T1."Run Time System" ("Application:Kind")) -> (x = y?=w255:bool)
            n84 = call <userlib>:"Get Debug Mode.vi"("error in (no error)"=w250, "SMO"=w261) -> ("error out"=w251:errorcluster, "Behavior"=w260:T7)  [unwired: 7 in, 1 out]
            n85 = case shown="\"Normal\", Default" w260 {
              tunnel: [w265 w267] -> w257
              tunnel: w256 -> [w265 _]
              tunnel: w255 -> [_ w269]
              tunnel: [_ "UI: Front Panel State >> Open\nUI: Wait >> 1000"] -> w254
              frame "Normal", Default {
                # "respect core.close"
              }
              frame "Debug" {
                # "keep panel open\nunless exe"
                n86 = Or(x=w269, y=FALSE) -> (x .or. y?=w267:bool)
              }
            }
            n87 = Bundle By Name(cluster=w252, "Core.Close Panel on Exit?"=w257) -> (w253:T4)
            n88 = call <vilib>:"Add State(s) to Queue__jki_lib_state_machine.vi"("State(s) in Front (\"\")"=w254, "State(s) in (\"\")"=w264) -> ("States Out"=w263:string)  [unwired: 13 in]
          }
          frame "Macro: Exit" {
            # "Exit Macro\n(This is called once, when the VI exits)"
            n89 = Unbundle By Name(w270) -> ("Core.Close Panel on Exit?"=w282:bool)
            n90 = Bundle By Name(cluster=w270, "Core.Shutdown?"=TRUE) -> (w271:T4)
            n91 = Select(t="UI: Front Panel State >> Close", s=w282, f="") -> (s? t:f=w279:string)
            n92 = call <vilib>:"Add State(s) to Queue__jki_lib_state_machine.vi"("State(s) in Front (\"\")"="VRM: Close\nData: Cleanup\nEvents: Unregister", "State(s) in (\"\")"="Process: Sync", "State(s) at Back (\"\")"="Exit") -> ("States Out"=w274:string)  [unwired: 12 in]
            n93 = call <vilib>:"Add State(s) to Queue__jki_lib_state_machine.vi"("State(s) in (\"\")"=w279, "State(s) at Back (\"\")"=w274) -> ("States Out"=w278:string)  [unwired: 13 in]
            n94 = call <vilib>:"Add State(s) to Queue__jki_lib_state_machine.vi"("State(s) in Front (\"\")"=w278, "State(s) in (\"\")"=w285) -> ("States Out"=w284:string)  [unwired: 13 in]
          }
          frame "Macro: Run Sequence" {
            # "0,1,2,3,4,"
            # "5"
            # "Do not put any code in this frame.\n(It is a separator no-op. You can make a copy of this frame to create a new Macro frame)"
            n95 = Unbundle By Name(w290) -> ("sequence"=w296:string[], "Running Step"=w288:i32)
            n96 = Index Array(array=w296, index=w288) -> (element=w294:string)
            n97 = Array Size(array=w296) -> (size(s)=w297:i32)
            n98 = Equal?(x=w297, y=w288) -> (x = y?=w289:bool)
            n99 = Select(t=-1 ("Running Step"), s=w289, f=w288) -> (s? t:f=w295:i32)
            n100 = Select(t="Sequence: Update Status >> ...", s=w289, f="Idle\nMacro: Run Sequence" ("State(s) at Back (\"\")")) -> (s? t:f=w291:string)
            n101 = Bundle By Name(cluster=w290, "Running Step"=w295) -> (w298:T4)
            n102 = call <vilib>:"Add State(s) to Queue__jki_lib_state_machine.vi"("State(s) in Front (\"\")"=w294, "State(s) at Back (\"\")"=w291) -> ("States Out"=w293:string)  [unwired: 13 in]
            n103 = call <vilib>:"Add State(s) to Queue__jki_lib_state_machine.vi"("State(s) in Front (\"\")"=w293, "State(s) in (\"\")"=w302) -> ("States Out"=w301:string)  [unwired: 13 in]
          }
          frame "Macro: Load SetMagnet Sequence" {
            # "PUT IN HOLD\nUPDATE TARGET\nRAMP TO TARGET\nCHECK HOLD"
            # "clear the queue"
            n104 = Unbundle By Name(w312) -> ("SelfRef"=w311:refnum<class "Instrument.OxfordVRM.lvclass">, "Field (T)"=w307:dbl[], "Axis"=w303:T3)
            n105 = call "Get Field.vi"("Axis"=VRM_Magnet_Axis--Enum."ALL", "error in (no error)"=w310, "Instrument.VRM in"=w311) -> ("error out"=w309:errorcluster, "Field (T)"=w308:dbl[])  [unwired: 6 in, 1 out]
            n106 = case shown="\"ALL\"" w303 {
              tunnel: w308 -> [w321 w325 w331 w337]
              tunnel: w307 -> [w320 w326 w332 w338]
              tunnel: [w319 w327 w333 w339] -> w306
              frame "ALL" {
                n107 = call "Instrument.OxfordVRM.FloatApprox (Array).vi"("y"=w320, "x"=w321) -> ("x ~ y?"=w319:bool)  [unwired: 4 in]
              }
              frame "Z" {
                n108 = Index Array(array=w325, index=2) -> (element=w323:dbl)
                n109 = Index Array(array=w326) -> (element=w324:dbl)  [unwired: 1 in]
                n110 = call "Instrument.OxfordVRM.FloatApprox.vi"("y"=w324, "x"=w323) -> ("x ~ y?"=w327:bool)  [unwired: 4 in]
              }
              frame "X" {
                n111 = Index Array(array=w331, index=0) -> (element=w329:dbl)
                n112 = Index Array(array=w332) -> (element=w330:dbl)  [unwired: 1 in]
                n113 = call "Instrument.OxfordVRM.FloatApprox.vi"("y"=w330, "x"=w329) -> ("x ~ y?"=w333:bool)  [unwired: 4 in]
              }
              frame "Y" {
                n114 = Index Array(array=w337, index=1) -> (element=w335:dbl)
                n115 = Index Array(array=w338) -> (element=w336:dbl)  [unwired: 1 in]
                n116 = call "Instrument.OxfordVRM.FloatApprox.vi"("y"=w336, "x"=w335) -> ("x ~ y?"=w339:bool)  [unwired: 4 in]
              }
            }
            n117 = call <userlib>:"String to 1D Array__ogtk.vi"("delimiter (Tab)"="\n", "string"="VRM: Hold\nSequence: Check Hold\nVRM: Set Target\nSequence: Check Targets Match\nVRM: RTOS\nSequence: Check Hold" ("State(s) in Front (\"\")")) -> ("Array of Strings"=w316:string[])  [unwired: 9 in]
            n118 = case shown="False" w306 {
              tunnel: w316 -> [w343 _]
              tunnel: ["Macro: Run Sequence" ("State(s) in Front (\"\")") "" ("State(s) in Front (\"\")")] -> w315
              tunnel: [w341 w345] -> w313
              tunnel: w312 -> [w340 w345]
              frame False {
                n119 = Bundle By Name(cluster=w340, "Running Step"=0 ("sequence"), "sequence"=w343) -> (w341:T4)
              }
              frame True {
              }
            }
            n120 = call <vilib>:"Add State(s) to Queue__jki_lib_state_machine.vi"("State(s) in Front (\"\")"=w315) -> ("States Out"=w318:string)  [unwired: 14 in]
          }
          frame "Macro: Abort Sequence" {
            n121 = call <userlib>:"String to 1D Array__ogtk.vi"("delimiter (Tab)"="\n", "string"="" ("State(s) in Front (\"\")")) -> ("Array of Strings"=w354:string[])  [unwired: 9 in]
            n122 = Bundle By Name(cluster=w350, "Running Step"=0 ("sequence"), "sequence"=w354) -> (w351:T4)
            n123 = call <vilib>:"Add State(s) to Queue__jki_lib_state_machine.vi"("State(s) in Front (\"\")"="Macro: Run Sequence" ("State(s) in Front (\"\")")) -> ("States Out"=w356:string)  [unwired: 14 in]
          }
          frame "---------- Process ----------" {
            # "Template Separator\n(You can make a copy of, or modify, this frame)"
            n124 = call <vilib>:"Add State(s) to Queue__jki_lib_state_machine.vi"("State(s) in (\"\")"=w361) -> ("States Out"=w360:string)  [unwired: 14 in]
          }
          frame "Process: Sync" {
            n125 = Unbundle By Name(w362) -> ("SelfRef"=w366:refnum<class "Instrument.OxfordVRM.lvclass">)
            n126 = call <vilib>:"WaitOnProcessSync.vi"("error in (no error)"=w365, "SMO"=w366) -> ("error out"=w364:errorcluster, "Don't run?"=w369:bool)  [unwired: 7 in, 1 out]
            n127 = Select(t="Data: Cleanup\nEvents: Unregister\nExit", s=w369, f="") -> (s? t:f=w363:string)
            n128 = call <vilib>:"Add State(s) to Queue__jki_lib_state_machine.vi"("State(s) in Front (\"\")"=w363, "State(s) in (\"\")"=w372) -> ("States Out"=w371:string)  [unwired: 13 in]
          }
          frame "---------- Events ----------" {
            # "Template Separator\n(You can make a copy of, or modify, this frame)"
            n129 = call <vilib>:"Add State(s) to Queue__jki_lib_state_machine.vi"("State(s) in (\"\")"=w377) -> ("States Out"=w376:string)  [unwired: 14 in]
          }
          frame "Events: Register" {
            # "Expand to add\nmore events"
            n130 = Unbundle By Name(w388) -> ("SelfRef"=w385:refnum<class "Instrument.OxfordVRM.lvclass">)
            n131 = call <vilib>:"GetProtectedEvents.vi"("SMO"=w385) -> ("error out"=w381:errorcluster, "SMO Protected Events"=w386:T8, "SMO out"=w380:refnum<class "Instrument.OxfordVRM.lvclass">)  [unwired: 8 in]
            n132 = call "Instrument.OxfordVRM.GetPrivateEvents.vi"("Instrument.Oxford1820"=w380) -> ("error out"=w379:errorcluster, "Instrument.VRM.Private Events"=w378:T9)  [unwired: 8 in, 1 out]
            n133 = register-events(w386, w378) -> (reference out=w387:refnum<event-registration>, error out=w382:errorcluster)  [unwired: 2 in]
            n134 = Merge Errors(w379, w384, w382, w381) -> (w383:errorcluster)
            n135 = call <vilib>:"Add State(s) to Queue__jki_lib_state_machine.vi"("State(s) in (\"\")"=w390) -> ("States Out"=w389:string)  [unwired: 14 in]
          }
          frame "Events: Unregister" {
            n136 = Unregister For Events(event registration refnum=w393, error in=w392) -> (error out=w391:errorcluster)
            n137 = call <vilib>:"Clear Errors.vi"("error in (no error)"=w391) -> ()  [unwired: 5 in, 2 out]
            n138 = call <vilib>:"Add State(s) to Queue__jki_lib_state_machine.vi"("State(s) in (\"\")"=w396) -> ("States Out"=w395:string)  [unwired: 14 in]
          }
          frame "---------- Sequence ----------" {
            n139 = Unbundle By Name(w397) -> ("Running Step"=w398:i32, "SelfRef"=w401:refnum<class "Instrument.OxfordVRM.lvclass">)
            n140 = Increment(x=w398) -> (x+1=w400:i32)
            n141 = Bundle By Name(cluster=w397, "Running Step"=w400, "SelfRef"=w401) -> (w399:T4)
            n142 = call <vilib>:"Add State(s) to Queue__jki_lib_state_machine.vi"("State(s) in (\"\")"=w405) -> ("States Out"=w404:string)  [unwired: 14 in]
          }
          frame "Sequence: Template" {
            n143 = Unbundle By Name(w408) -> ("SelfRef"=w406:refnum<class "Instrument.OxfordVRM.lvclass">)
            n144 = Bundle By Name(cluster=w408, "SelfRef"=w406) -> (w407:T4)
            n145 = call <vilib>:"Add State(s) to Queue__jki_lib_state_machine.vi"("State(s) in (\"\")"=w412) -> ("States Out"=w411:string)  [unwired: 14 in]
          }
          frame "Sequence: Wait" {
            # "F = repeat this state. wait\nT = go to next state. don't wait"
            n146 = Unbundle By Name(w415) -> ("Running Step"=w438:i32)
            n147 = Equal?(x=w430, y="RESET") -> (x = y?=w434:bool)
            n148 = case shown="False" w434 {
              tunnel: [w443 u32 10000 ("time (ms)")] -> w433
              tunnel: [w446 w448] -> w420
              tunnel: w418 -> [w445 w448]
              tunnel: w430 -> [w444 _]
              frame False {
                n149 = Scan From String(format string="%d", input string=w444, error in=w445) -> (error out=w446:errorcluster, output 1=w442:i32)  [unwired: 2 in, 2 out]
                n150 = To Unsigned Long Integer(number=w442) -> (unsigned 32bit integer=w443:u32)
              }
              frame True {
              }
            }
            n151 = call <userlib>:"Periodic Trigger__ogtk.vi"("time (ms)"=w433, "reset"=w434) -> ("Triggered"=w435:bool, "timer value"=w432:u32)  [unwired: 11 in, 1 out]
            n152 = Or(x=w435, y=w434) -> (x .or. y?=w417:bool)
            n153 = Increment(x=w438) -> (x+1=w437:i32)
            n154 = Subtract(x=w433, y=w432) -> (x-y=w424:u32)
            "timer" <- w424
            n155 = Select(t=u32 0, s=w417, f=u32 100 ("milliseconds to wait")) -> (s? t:f=w422:u32)
            n156 = Select(t=w437, s=w417, f=w438) -> (s? t:f=w436:i32)
            n157 = call <userlib>:"Wait (ms)__ogtk.vi"("error in (no error)"=w420, "milliseconds to wait"=w422) -> ("error out"=w419:errorcluster)  [unwired: 8 in, 1 out]
            n158 = Bundle By Name(cluster=w415, "Running Step"=w436) -> (w413:T4)
            n159 = Divide(x=w424, y=u32 1000) -> (x/y=w426:dbl)
            n160 = Format Into String(format string="%s >> %d s", w429, w426) -> (resulting string=w427:string)  [unwired: 2 in, 1 out]
            n161 = call <vilib>:"Build State String with Arguments__JKI_lib_State_Machine.vi"("Arguments (\"\")"=w427, "State"="Sequence: Update Status") -> ("State with Arguments"=w414:string)  [unwired: 4 in]
            n162 = call <vilib>:"Add State(s) to Queue__jki_lib_state_machine.vi"("State(s) in Front (\"\")"=w414, "State(s) in (\"\")"=w441) -> ("States Out"=w440:string)  [unwired: 13 in]
          }
          frame "Sequence: Update Status" {
            n163 = Unbundle By Name(w451) -> ("SelfRef"=w456:refnum<class "Instrument.OxfordVRM.lvclass">)
            n164 = call "Instrument.OxfordVRM.ProcessStatus.vi"("error in (no error)"=w455, "event data"=w452, "Instrument.Oxford1820"=w456) -> ("error out"=w454:errorcluster, "Instrument.Oxford1820 out"=w453:refnum<class "Instrument.OxfordVRM.lvclass">)  [unwired: 7 in]
            n165 = Bundle By Name(cluster=w451, "SelfRef"=w453) -> (w450:T4)
            n166 = call <vilib>:"Add State(s) to Queue__jki_lib_state_machine.vi"("State(s) in (\"\")"=w459) -> ("States Out"=w458:string)  [unwired: 14 in]
          }
          frame "Sequence: Check Hold" {
            # "F = repeat this state. wait\nT = go to next state. don't wait"
            n167 = Unbundle By Name(w474) -> ("Running Step"=w476:i32, "SelfRef"=w470:refnum<class "Instrument.OxfordVRM.lvclass">, "Axis"=w460:T3)
            n168 = call "Get Status.vi"("Axis"=w460, "error in (no error)"=w462, "Instrument.VRM in"=w470) -> ("error out"=w464:errorcluster, "Status (ALL)"=w478:T10, "Instrument.VRM out"=w461:refnum<class "Instrument.OxfordVRM.lvclass">)  [unwired: 5 in, 1 out]
            n169 = Unbundle By Name(w478) -> ("Holding"=w465:bool)
            n170 = Increment(x=w476) -> (x+1=w477:i32)
            n171 = Select(t=w477, s=w465, f=w476) -> (s? t:f=w475:i32)
            n172 = Select(t=u32 0, s=w465, f=u32 500 ("milliseconds to wait")) -> (s? t:f=w467:u32)
            n173 = Bundle By Name(cluster=w474, "Running Step"=w475, "SelfRef"=w461) -> (w473:T4)
            n174 = call <userlib>:"Wait (ms)__ogtk.vi"("error in (no error)"=w464, "milliseconds to wait"=w467) -> ("error out"=w463:errorcluster)  [unwired: 8 in, 1 out]
            n175 = call <vilib>:"Build State String with Arguments__JKI_lib_State_Machine.vi"("Arguments (\"\")"=w471, "State"="Sequence: Update Status") -> ("State with Arguments"=w469:string)  [unwired: 4 in]
            n176 = call <vilib>:"Add State(s) to Queue__jki_lib_state_machine.vi"("State(s) in Front (\"\")"=w469, "State(s) in (\"\")"=w481) -> ("States Out"=w480:string)  [unwired: 13 in]
          }
          frame "Sequence: Check RTOS" {
            # "F = repeat this state. wait\nT = go to next state. don't wait"
            n177 = Unbundle By Name(w496) -> ("Running Step"=w498:i32, "SelfRef"=w492:refnum<class "Instrument.OxfordVRM.lvclass">, "Axis"=w482:T3)
            n178 = call "Get Status.vi"("Axis"=w482, "error in (no error)"=w484, "Instrument.VRM in"=w492) -> ("error out"=w486:errorcluster, "Status (ALL)"=w500:T10, "Instrument.VRM out"=w483:refnum<class "Instrument.OxfordVRM.lvclass">)  [unwired: 5 in, 1 out]
            n179 = Unbundle By Name(w500) -> ("Ramp to Setpoint"=w487:bool)
            n180 = Increment(x=w498) -> (x+1=w499:i32)
            n181 = Select(t=w499, s=w487, f=w498) -> (s? t:f=w497:i32)
            n182 = Select(t=u32 0, s=w487, f=u32 500 ("milliseconds to wait")) -> (s? t:f=w489:u32)
            n183 = Bundle By Name(cluster=w496, "Running Step"=w497, "SelfRef"=w483) -> (w495:T4)
            n184 = call <userlib>:"Wait (ms)__ogtk.vi"("error in (no error)"=w486, "milliseconds to wait"=w489) -> ("error out"=w485:errorcluster)  [unwired: 8 in, 1 out]
            n185 = call <vilib>:"Build State String with Arguments__JKI_lib_State_Machine.vi"("Arguments (\"\")"=w493, "State"="Sequence: Update Status") -> ("State with Arguments"=w491:string)  [unwired: 4 in]
            n186 = call <vilib>:"Add State(s) to Queue__jki_lib_state_machine.vi"("State(s) in Front (\"\")"=w491, "State(s) in (\"\")"=w503) -> ("States Out"=w502:string)  [unwired: 13 in]
          }
          frame "Sequence: Check RTOZ" {
            # "F = repeat this state. wait\nT = go to next state. don't wait"
            n187 = Unbundle By Name(w518) -> ("Running Step"=w520:i32, "SelfRef"=w514:refnum<class "Instrument.OxfordVRM.lvclass">, "Axis"=w504:T3)
            n188 = call "Get Status.vi"("Axis"=w504, "error in (no error)"=w506, "Instrument.VRM in"=w514) -> ("error out"=w508:errorcluster, "Status (ALL)"=w522:T10, "Instrument.VRM out"=w505:refnum<class "Instrument.OxfordVRM.lvclass">)  [unwired: 5 in, 1 out]
            n189 = Unbundle By Name(w522) -> ("Ramp to Zero"=w509:bool)
            n190 = Increment(x=w520) -> (x+1=w521:i32)
            n191 = Select(t=w521, s=w509, f=w520) -> (s? t:f=w519:i32)
            n192 = Bundle By Name(cluster=w518, "Running Step"=w519, "SelfRef"=w505) -> (w517:T4)
            n193 = Select(t=u32 0, s=w509, f=u32 500 ("milliseconds to wait")) -> (s? t:f=w511:u32)
            n194 = call <userlib>:"Wait (ms)__ogtk.vi"("error in (no error)"=w508, "milliseconds to wait"=w511) -> ("error out"=w507:errorcluster)  [unwired: 8 in, 1 out]
            n195 = call <vilib>:"Build State String with Arguments__JKI_lib_State_Machine.vi"("Arguments (\"\")"=w515, "State"="Sequence: Update Status") -> ("State with Arguments"=w513:string)  [unwired: 4 in]
            n196 = call <vilib>:"Add State(s) to Queue__jki_lib_state_machine.vi"("State(s) in Front (\"\")"=w513, "State(s) in (\"\")"=w525) -> ("States Out"=w524:string)  [unwired: 13 in]
          }
          frame "Sequence: Check PSU at Zero" {
            # "#todo\nnot needed???"
            # "F = repeat this state. wait\nT = go to next state. don't wait"
            n197 = Unbundle By Name(w545) -> ("Running Step"=w542:i32, "SelfRef"=w537:refnum<class "Instrument.OxfordVRM.lvclass">, "Axis"=w526:T3)
            n198 = call "Get Field.vi"("Axis"=w526, "error in (no error)"=w532, "Instrument.VRM in"=w537) -> ("error out"=w531:errorcluster, "Field (T)"=w527:dbl[], "Instrument.VRM out"=w528:refnum<class "Instrument.OxfordVRM.lvclass">)  [unwired: 6 in]
            n199 = call "Instrument.OxfordVRM.FloatApprox (Array).vi"("y"=dbl[] [0.0, 0.0, 0.0], "x"=w527) -> ("x ~ y?"=w533:bool)  [unwired: 4 in]
            n200 = Increment(x=w542) -> (x+1=w543:i32)
            n201 = Select(t=w543, s=w533, f=w542) -> (s? t:f=w541:i32)
            n202 = Bundle By Name(cluster=w545, "Running Step"=w541, "SelfRef"=w528) -> (w544:T4)
            n203 = Select(t=u32 0, s=w533, f=u32 500 ("milliseconds to wait")) -> (s? t:f=w535:u32)
            n204 = call <userlib>:"Wait (ms)__ogtk.vi"("error in (no error)"=w531, "milliseconds to wait"=w535) -> ("error out"=w530:errorcluster)  [unwired: 8 in, 1 out]
            n205 = call <vilib>:"Build State String with Arguments__JKI_lib_State_Machine.vi"("Arguments (\"\")"=w538, "State"="Sequence: Update Status") -> ("State with Arguments"=w539:string)  [unwired: 4 in]
            n206 = call <vilib>:"Add State(s) to Queue__jki_lib_state_machine.vi"("State(s) in Front (\"\")"=w539, "State(s) in (\"\")"=w548) -> ("States Out"=w547:string)  [unwired: 13 in]
          }
          frame "Sequence: Check Targets Match" {
            # "F = repeat this state. wait\nT = go to next state. don't wait"
            n207 = Unbundle By Name(w568) -> ("Running Step"=w565:i32, "SelfRef"=w557:refnum<class "Instrument.OxfordVRM.lvclass">, "Field (T)"=w550:dbl[], "Axis"=w549:T3)
            n208 = call "Get Target.vi"("Axis"=w549, "error in (no error)"=w556, "Instrument.VRM in"=w557) -> ("error out"=w555:errorcluster, "Target Field (T)"=w554:dbl[], "Instrument.VRM out"=w552:refnum<class "Instrument.OxfordVRM.lvclass">)  [unwired: 5 in, 1 out]
            n209 = call "Instrument.OxfordVRM.FloatApprox (Array).vi"("y"=w550, "x"=w554) -> ("x ~ y?"=w551:bool)  [unwired: 4 in]
            n210 = Increment(x=w565) -> (x+1=w566:i32)
            n211 = Select(t=w566, s=w551, f=w565) -> (s? t:f=w564:i32)
            n212 = Select(t=u32 0, s=w551, f=u32 500 ("milliseconds to wait")) -> (s? t:f=w559:u32)
            n213 = call <userlib>:"Wait (ms)__ogtk.vi"("error in (no error)"=w555, "milliseconds to wait"=w559) -> ("error out"=w561:errorcluster)  [unwired: 8 in, 1 out]
            n214 = Bundle By Name(cluster=w568, "Running Step"=w564, "SelfRef"=w552) -> (w567:T4)
            n215 = call <vilib>:"Build State String with Arguments__JKI_lib_State_Machine.vi"("Arguments (\"\")"=w562, "State"="Sequence: Update Status") -> ("State with Arguments"=w553:string)  [unwired: 4 in]
            n216 = call <vilib>:"Add State(s) to Queue__jki_lib_state_machine.vi"("State(s) in Front (\"\")"=w553, "State(s) in (\"\")"=w571) -> ("States Out"=w570:string)  [unwired: 13 in]
          }
          frame "---------- VRM ----------" {
            n217 = Unbundle By Name(w574) -> ("Running Step"=w572:i32, "SelfRef"=w576:refnum<class "Instrument.OxfordVRM.lvclass">)
            n218 = Increment(x=w572) -> (x+1=w575:i32)
            n219 = Bundle By Name(cluster=w574, "Running Step"=w575, "SelfRef"=w576) -> (w573:T4)
            n220 = call <vilib>:"Add State(s) to Queue__jki_lib_state_machine.vi"("State(s) in (\"\")"=w580) -> ("States Out"=w579:string)  [unwired: 14 in]
          }
          frame "VRM: Open" {
            n221 = Unbundle By Name(w586) -> ("SelfRef"=w585:refnum<class "Instrument.OxfordVRM.lvclass">)
            n222 = call-dynamic "Open Hardware.vi"("error in (no error)"=w582, "Instrument.VRM in"=w585) -> ("error out"=w583:errorcluster, "Instrument.VRM out"=w584:refnum<class "Instrument.OxfordVRM.lvclass">)  [unwired: 8 in]
            n223 = Bundle By Name(cluster=w586, "SelfRef"=w584) -> (w581:T4)
            n224 = call <vilib>:"Add State(s) to Queue__jki_lib_state_machine.vi"("State(s) in (\"\")"=w589) -> ("States Out"=w588:string)  [unwired: 14 in]
          }
          frame "VRM: Close" {
            n225 = Unbundle By Name(w595) -> ("SelfRef"=w594:refnum<class "Instrument.OxfordVRM.lvclass">)
            n226 = call-dynamic "Close Hardware.vi"("error in (no error)"=w591, "Instrument.VRM in"=w594) -> ("error out"=w592:errorcluster, "Instrument.VRM out"=w593:refnum<class "Instrument.OxfordVRM.lvclass">)  [unwired: 8 in]
            n227 = Bundle By Name(cluster=w595, "SelfRef"=w593) -> (w590:T4)
            n228 = call <vilib>:"Add State(s) to Queue__jki_lib_state_machine.vi"("State(s) in (\"\")"=w598) -> ("States Out"=w597:string)  [unwired: 14 in]
          }
          frame "VRM: GetAll" {
            n229 = Unbundle By Name(w605) -> ("SelfRef"=w607:refnum<class "Instrument.OxfordVRM.lvclass">)
            n230 = call "Read IPS All.vi"("error in (no error)"=w604, "Instrument.VRM in"=w607) -> ("error out"=w600:errorcluster, "output cluster"=w602:T6, "Instrument.VRM out"=w603:refnum<class "Instrument.OxfordVRM.lvclass">)  [unwired: 7 in]
            n231 = call <userlib>:"setAllData.vi"("error in (no error)"=w600, "AllData"=w602, "Instrument in"=w603) -> ("error out"=w599:errorcluster, "Instrument out"=w601:refnum<class "Instrument.OxfordVRM.lvclass">)  [unwired: 7 in]
            n232 = Bundle By Name(cluster=w605, "SelfRef"=w601) -> (w606:T4)
            n233 = call <vilib>:"Add State(s) to Queue__jki_lib_state_machine.vi"("State(s) in (\"\")"=w610) -> ("States Out"=w609:string)  [unwired: 14 in]
          }
          frame "VRM: Hold" {
            n234 = Unbundle By Name(w622) -> ("Running Step"=w615:i32, "SelfRef"=w611:refnum<class "Instrument.OxfordVRM.lvclass">, "Axis"=w612:T3)
            n235 = Increment(x=w615) -> (x+1=w614:i32)
            n236 = call "Hold.vi"("Axis"=w612, "error in (no error)"=w613, "Instrument.VRM in"=w611) -> ("error out"=w619:errorcluster, "Instrument.VRM out"=w620:refnum<class "Instrument.OxfordVRM.lvclass">)  [unwired: 6 in, 1 out]
            n237 = Bundle By Name(cluster=w622, "Running Step"=w614, "SelfRef"=w620) -> (w621:T4)
            n238 = call <vilib>:"Build State String with Arguments__JKI_lib_State_Machine.vi"("Arguments (\"\")"=w616, "State"="Sequence: Update Status") -> ("State with Arguments"=w618:string)  [unwired: 4 in]
            n239 = call <vilib>:"Add State(s) to Queue__jki_lib_state_machine.vi"("State(s) in Front (\"\")"=w618, "State(s) in (\"\")"=w625) -> ("States Out"=w624:string)  [unwired: 13 in]
          }
          frame "VRM: RTOS" {
            n240 = Unbundle By Name(w637) -> ("Running Step"=w628:i32, "SelfRef"=w630:refnum<class "Instrument.OxfordVRM.lvclass">, "Axis"=w626:T3)
            n241 = Increment(x=w628) -> (x+1=w627:i32)
            n242 = call "Ramp to Set.vi"("Axis"=w626, "error in (no error)"=w629, "Instrument.VRM in"=w630) -> ("error out"=w634:errorcluster, "Instrument.VRM out"=w635:refnum<class "Instrument.OxfordVRM.lvclass">)  [unwired: 6 in, 1 out]
            n243 = Bundle By Name(cluster=w637, "Running Step"=w627, "SelfRef"=w635) -> (w636:T4)
            n244 = call <vilib>:"Build State String with Arguments__JKI_lib_State_Machine.vi"("Arguments (\"\")"=w631, "State"="Sequence: Update Status") -> ("State with Arguments"=w633:string)  [unwired: 4 in]
            n245 = call <vilib>:"Add State(s) to Queue__jki_lib_state_machine.vi"("State(s) in Front (\"\")"=w633, "State(s) in (\"\")"=w640) -> ("States Out"=w639:string)  [unwired: 13 in]
          }
          frame "VRM: RTOZ" {
            # "#todo: add abort public method"
            # "#todo: make these separate states\n1. check B = Target?\n2. Turn on switch\n3. set PSU to target\n4. check hold OR psu = target\n5. set persist mode"
            n246 = Unbundle By Name(w652) -> ("Running Step"=w650:i32, "SelfRef"=w645:refnum<class "Instrument.OxfordVRM.lvclass">, "Axis"=w641:T3)
            n247 = call "Ramp to Zero.vi"("Axis"=w641, "error in (no error)"=w644, "Instrument.VRM in"=w645) -> ("error out"=w643:errorcluster, "Instrument.VRM out"=w642:refnum<class "Instrument.OxfordVRM.lvclass">)  [unwired: 6 in, 1 out]
            n248 = Increment(x=w650) -> (x+1=w649:i32)
            n249 = Bundle By Name(cluster=w652, "Running Step"=w649, "SelfRef"=w642) -> (w651:T4)
            n250 = call <vilib>:"Build State String with Arguments__JKI_lib_State_Machine.vi"("Arguments (\"\")"=w647, "State"="Sequence: Update Status") -> ("State with Arguments"=w646:string)  [unwired: 4 in]
            n251 = call <vilib>:"Add State(s) to Queue__jki_lib_state_machine.vi"("State(s) in Front (\"\")"=w646, "State(s) in (\"\")"=w655) -> ("States Out"=w654:string)  [unwired: 13 in]
          }
          frame "VRM: Set Target" {
            n252 = Unbundle By Name(w669) -> ("Running Step"=w667:i32, "SelfRef"=w663:refnum<class "Instrument.OxfordVRM.lvclass">, "Field (T)"=w662:dbl[], "Field Rate (T/min)"=w661:dbl, "Axis"=w656:T3)
            n253 = Increment(x=w667) -> (x+1=w666:i32)
            n254 = call "Set Target.vi"("Axis"=w656, "error in (no error)"=w660, "Target Rate Limit (T/min)"=w661, "Target Field (T)"=w662, "Instrument.VRM in"=w663) -> ("error out"=w659:errorcluster, "Instrument.VRM out"=w658:refnum<class "Instrument.OxfordVRM.lvclass">)  [unwired: 5 in]
            n255 = Bundle By Name(cluster=w669, "Running Step"=w666, "SelfRef"=w658) -> (w668:T4)
            n256 = call <vilib>:"Build State String with Arguments__JKI_lib_State_Machine.vi"("Arguments (\"\")"=w664, "State"="Sequence: Update Status") -> ("State with Arguments"=w665:string)  [unwired: 4 in]
            n257 = call <vilib>:"Add State(s) to Queue__jki_lib_state_machine.vi"("State(s) in Front (\"\")"=w665, "State(s) in (\"\")"=w672) -> ("States Out"=w671:string)  [unwired: 13 in]
          }
        }
      }
    }
    frame Error {
    }
  }
  n258 = call-parent "Process.vi"("error in"=w5, "Instrument"=w4) -> ("error out"=w2:errorcluster, "Instrument out"=→"Instrument.Example out":refnum<class "Instrument.OxfordVRM.lvclass">)  [unwired: 8 in]
  n259 = Merge Errors(w2, w1) -> (→"error out":errorcluster)
